vi "Array.vi"() -> ()   [LabVIEW 2022 SP3]
panel:
  out "subarray 2":dbl[](array[numeric])
  out "element":dbl
  out "appended array 2":dbl[][](array[numeric])
  out "appended array":dbl[](array[numeric])
  out "subarray":dbl[](array[numeric])
  out "size(s) 2":i32[](array[numeric])
  out "size(s)":i32
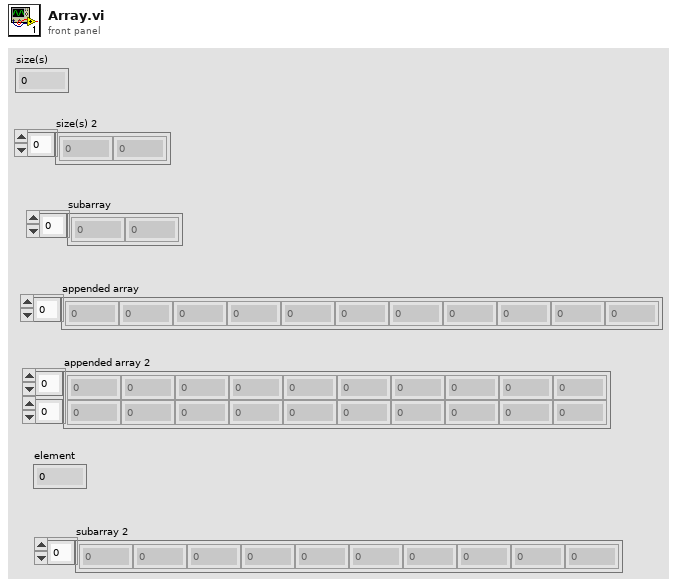
[diagram p1: front panel]
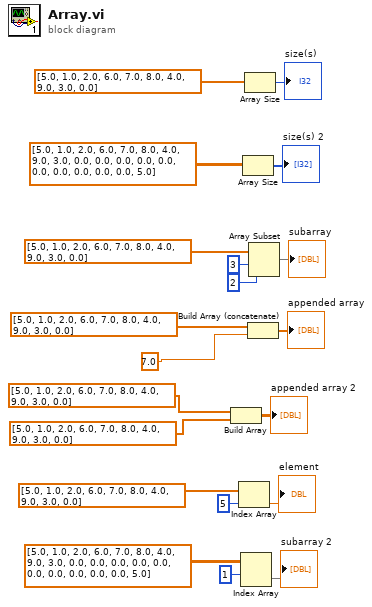
[diagram p0: block diagram]
diagram:
  n1 = Build Array(dbl[] [5.0, 1.0, 2.0, 6.0, 7.0, 8.0, 4.0, 9.0, 3.0, 0.0], dbl[] [5.0, 1.0, 2.0, 6.0, 7.0, 8.0, 4.0, 9.0, 3.0, 0.0]) -> (→"appended array 2":dbl[][])
  n2 = Index Array(array=dbl[] [5.0, 1.0, 2.0, 6.0, 7.0, 8.0, 4.0, 9.0, 3.0, 0.0], index=5) -> (element=→"element":dbl)
  n3 = Index Array(array=dbl[][] [[5.0, 1.0, 2.0, 6.0, 7.0, 8.0, 4.0, 9.0, 3.0, 0.0], [0.0, 0.0, 0.0, 0.0, 0.0, 0.0, 0.0, 0.0, 0.0, 5.0]], index (row)=1) -> (element=→"subarray 2":dbl[])  [unwired: 1 in]
  n4 = Array Size(array=dbl[][] [[5.0, 1.0, 2.0, 6.0, 7.0, 8.0, 4.0, 9.0, 3.0, 0.0], [0.0, 0.0, 0.0, 0.0, 0.0, 0.0, 0.0, 0.0, 0.0, 5.0]]) -> (size(s)=→"size(s) 2":i32[])
  n5 = Array Size(array=dbl[] [5.0, 1.0, 2.0, 6.0, 7.0, 8.0, 4.0, 9.0, 3.0, 0.0]) -> (size(s)=→"size(s)":i32)
  n6 = Build Array (concatenate)(dbl[] [5.0, 1.0, 2.0, 6.0, 7.0, 8.0, 4.0, 9.0, 3.0, 0.0], 7.0) -> (→"appended array":dbl[])
  n7 = Array Subset(array=dbl[] [5.0, 1.0, 2.0, 6.0, 7.0, 8.0, 4.0, 9.0, 3.0, 0.0], index=3, length=2) -> (→"subarray":dbl[])
